vi "Untitled 5 (SubVI).vi"(9 "Numeric":dbl, 10 "Array":u16[][](array[numeric]), 11 "Array 2":u16[](array[numeric])) -> (2 "Pressure in Pa.":dbl, 3 "Waveform Chart 2":dbl(graph))   [LabVIEW 2016]
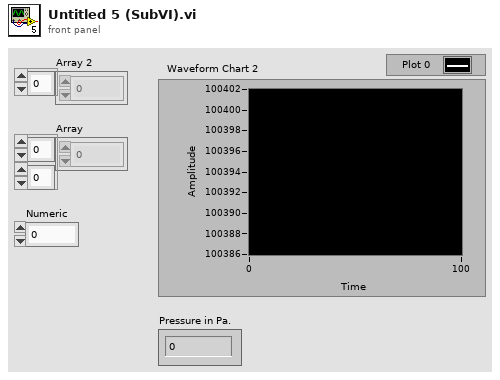
[diagram p1: front panel]
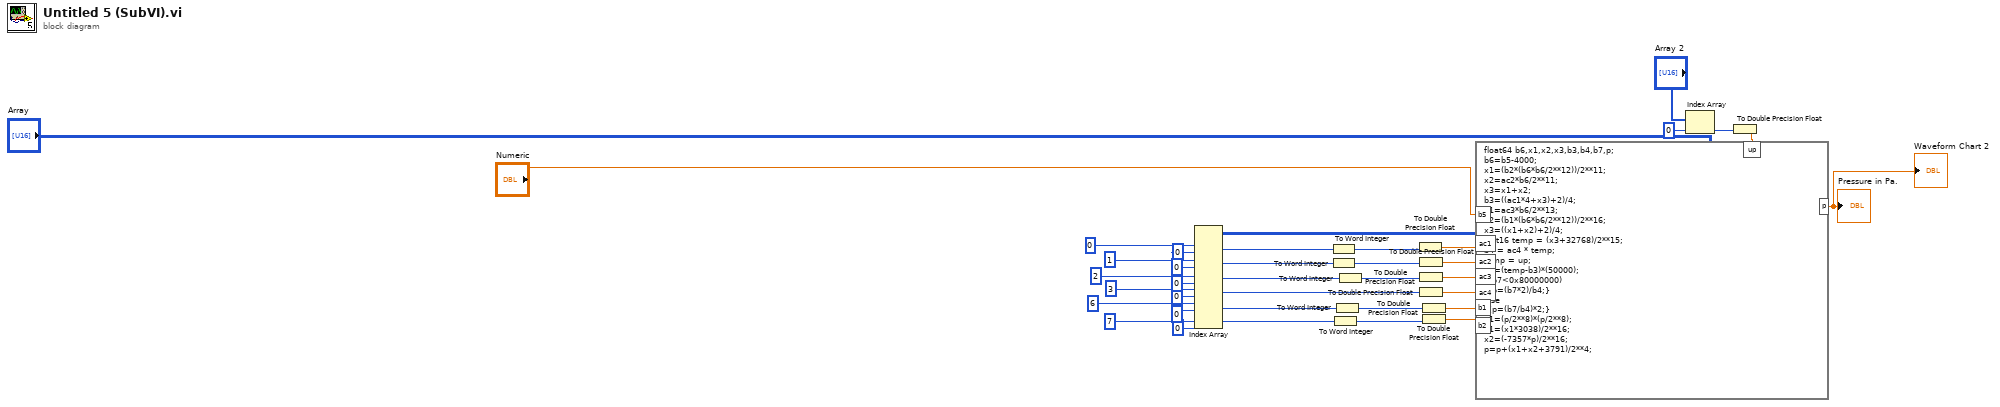
[diagram p0: block diagram]
diagram:
  n1 = Index Array(array="Array", index (row) #1=0 ("index (row)"), index (col) #1=0 ("index (col)"), index (row) #2=1 ("index (row)"), index (col) #2=0 ("index (col)"), index (row) #3=2 ("index (row)"), index (col) #3=0 ("index (col)"), index (row) #4=3 ("index (row)"), index (col) #4=0 ("index (col)"), index (row) #5=6 ("index (row)"), index (col) #5=0 ("index (col)"), index (row) #6=7 ("index (row)"), index (col) #6=0 ("index (col)")) -> (element #1=w28:u16, element #2=w30:u16, element #3=w31:u16, element #4=w32:u16, element #5=w33:u16, element #6=w34:u16)
  n2 = To Word Integer(number=w28) -> (16bit integer=w2:i16)
  n3 = To Word Integer(number=w30) -> (16bit integer=w35:i16)
  n4 = To Word Integer(number=w34) -> (16bit integer=w5:i16)
  n5 = To Word Integer(number=w33) -> (16bit integer=w4:i16)
  n6 = To Word Integer(number=w31) -> (16bit integer=w3:i16)
  n7 = To Double Precision Float(number=w2) -> (double precision float=w6:dbl)
  n8 = To Double Precision Float(number=w35) -> (double precision float=w36:dbl)
  n9 = To Double Precision Float(number=w3) -> (double precision float=w7:dbl)
  n10 = To Double Precision Float(number=w32) -> (double precision float=w8:dbl)
  n11 = To Double Precision Float(number=w4) -> (double precision float=w9:dbl)
  n12 = To Double Precision Float(number=w5) -> (double precision float=w10:dbl)
  n13 = Index Array(array="Array 2", index=0) -> (element=w13:u16)
  n14 = To Double Precision Float(number=w13) -> (double precision float=w14:dbl)
  n15 = formula code="float64 b6,x1,x2,x3,b3,b4,b7,p;\nb6=b5-4000;\nx1=(b2*(b6*b6/2**12))/2**11;\nx2=ac2*b6/2**11;\nx3=x1+x2;\nb3=((ac1*4+x3)+2)/4;\nx1=ac3*b6/2**13;\nx2=(b1*(b6*b6/2**12))/2**16;\nx3=((x1+x2)+2)/4;\nuInt16 temp = (x3+32768)/2**15;\nb4 = ac4 * temp;\ntemp = up;\nb7=(temp-b3)*(50000);\nif(b7<0x80000000)\n\t{p=(b7*2)/b4;}\nelse \n\t{p=(b7/b4)*2;}\nx1=(p/2**8)*(p/2**8);\nx1=(x1*3038)/2**16;\nx2=(-7357*p)/2**16;\np=p+(x1+x2+3791)/2**4;"("ac2"=w36, "ac3"=w7, "ac1"=w6, "b5"="Numeric", "up"=w14, "ac4"=w8, "b2"=w10, "b1"=w9) -> ("p"=→"Pressure in Pa." →"Waveform Chart 2":dbl)
